vi "Teeth Force Torque2___C.vi"() -> ()   [LabVIEW 2011]
doc: "Reads force and torque values from multiple ATI transducers."
uses:
  <vilib>/DAQmx/read.llb/DAQmx Read (Analog 2D DBL NChan NSamp).vi
  <vilib>/DAQmx/miscellaneous.llb/DAQmx Fill In Error Info.vi
  <vilib>/Analysis/baseanly.llb/A x Vector.vi
  <vilib>/Analysis/NI_AALBase.lvlib
  Program Files/MATLAB/R2010a/work/OSIM2/lib/OSIM_itf1.dll
panel:
  out "Average Voltages":dbl[][](array[numeric]) format="%#_3g"
  out "exiting":bool
  in  "stop":bool
  in  "Calibration File Directory:":path=path "C:/Documents and Settings/ortholab/Desktop/Load Cells Calibration Files Feb 2015"
  in  "Bias Transducer":bool[](array[boolean])=[FALSE, FALSE, FALSE, FALSE, FALSE, FALSE, FALSE, FALSE, FALSE, FALSE, FALSE, FALSE, FALSE, FALSE]
  in  "Calibration Files":string[](array[string])=["ft16995.cal", "ft6798.cal", "ft6799.cal", "ft6800.cal", "ft13847.cal", "ft6802.cal", "ft16994.cal", "ft6804.cal", "ft6805.cal", "ft5393.cal", "ft6807.cal", "ft6808.cal", "ft10276.cal", "ft13846.cal"]
  in  "Filename":path
  in  "Bias All":bool
  in  "Save Data Point":bool
  in  "Samples to Read at a time":i32=50
  out "Cal F/T Values":dbl[][](array[numeric])
  # "OSIM"
  # "Fx"
  # "Fy"
  # "Fz"
  # "Ty"
  # "Tz"
  # "Tx"
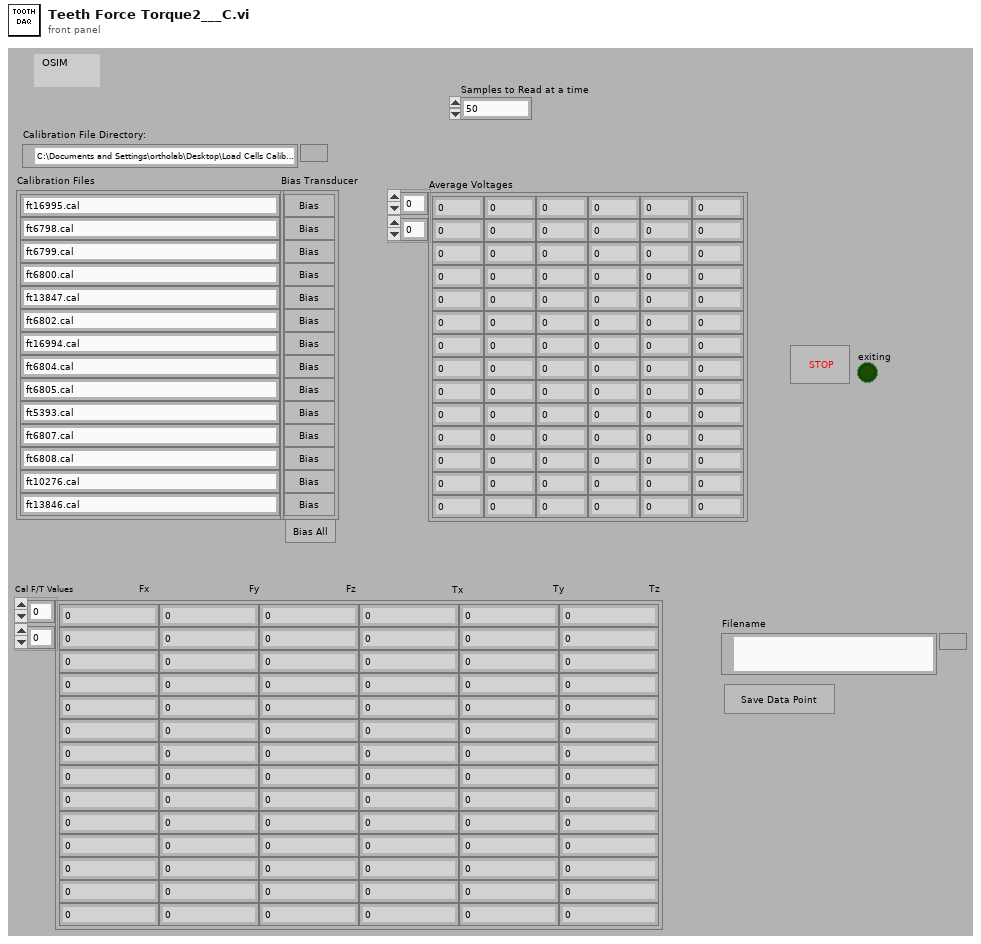
[diagram p1: front panel]
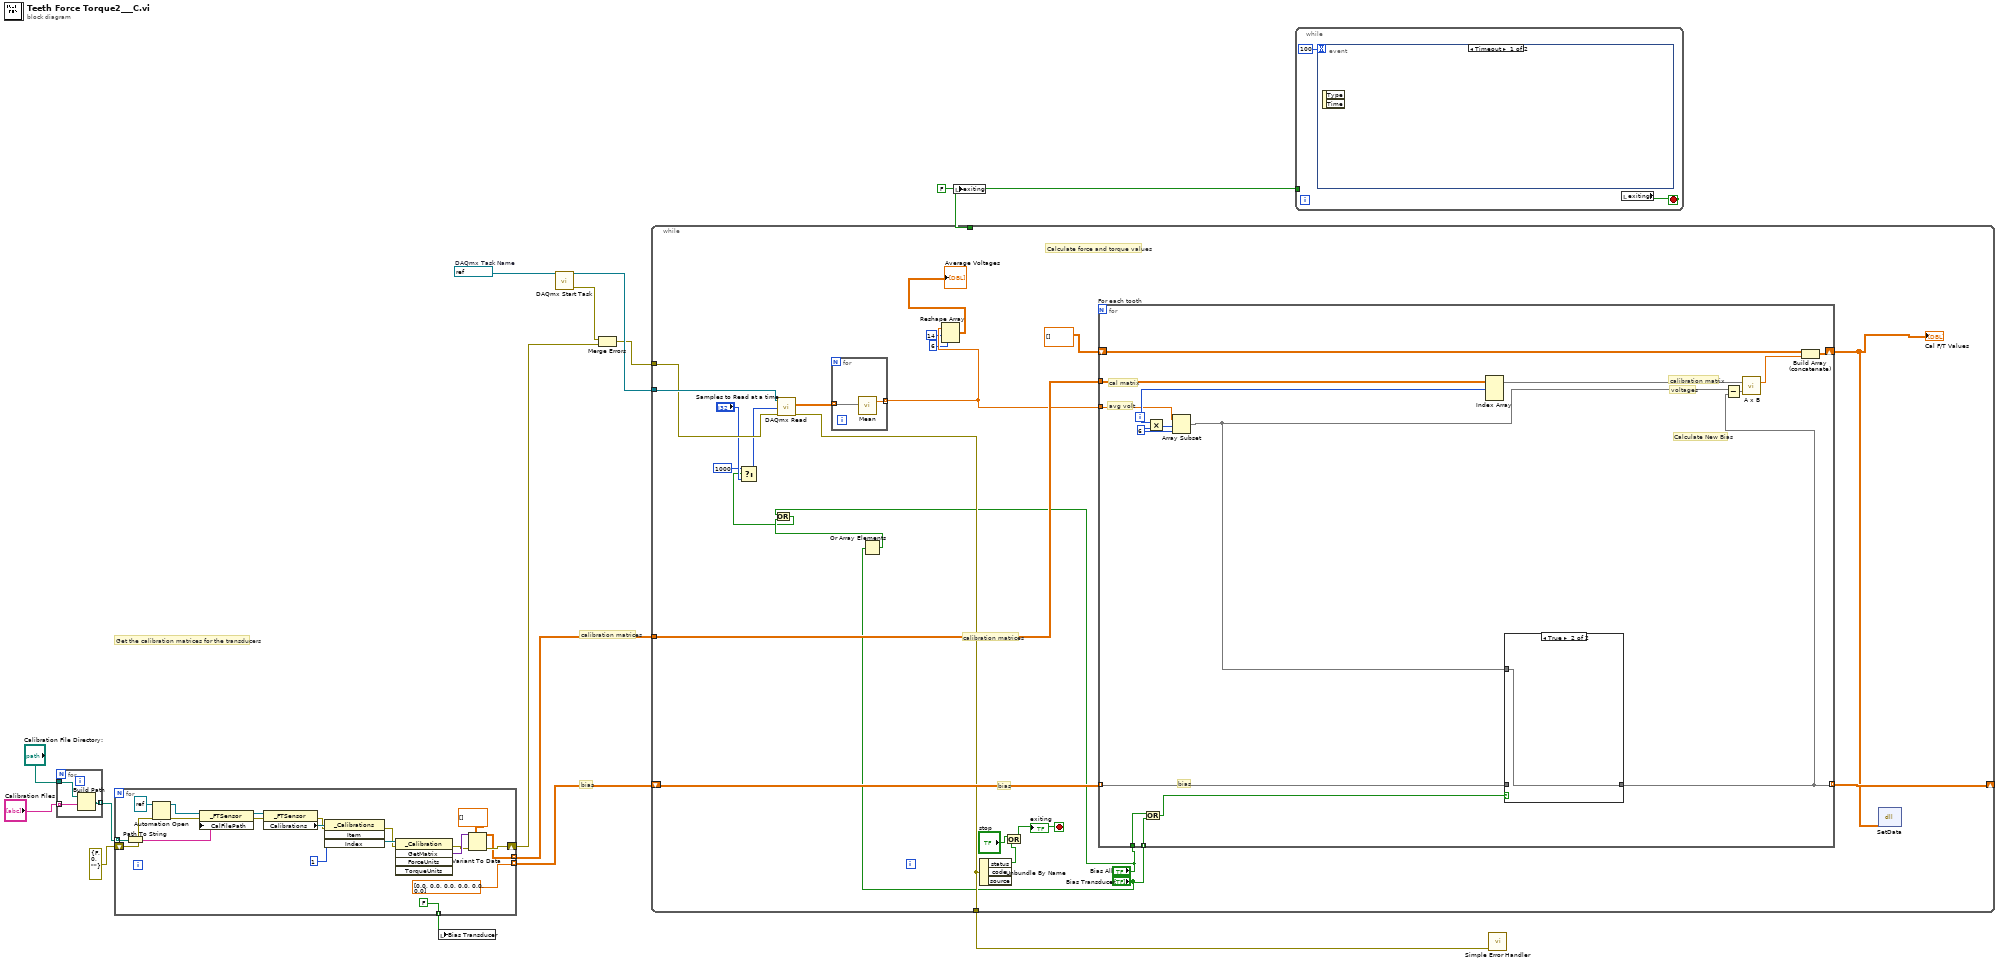
[diagram p0: block diagram]
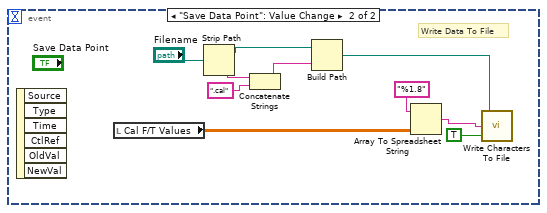
[diagram p2: hidden frame]
diagram:
  w1 = FALSE ("exiting")
  w2 = refnum<k21> "TEETH1"  # DAQmx Task Name
  # "bias"
  # "calibration matrices"
  # "Get the calibration matrices for the transducers"
  n1 = for {
    tunnel: "Calibration File Directory:" -> [w17]
    tunnel: [w16] -> w4 mode=indexing
    tunnel: "Calibration Files" -> [w15] mode=indexing
    n2 = Build Path(base path=w17, name or relative path=w15) -> (appended path=w16:path)
  }
  n3 = for {
    tunnel: w4 -> [w34] mode=indexing
    shift-right: [w25] -> w10
    shift-left: errorcluster {"status"=FALSE, "code"=0, "source"=""} ("error out") -> [w22]
    tunnel: [FALSE] -> w12 mode=indexing
    tunnel: [sgl[] [0.0, 0.0, 0.0, 0.0, 0.0, 0.0]] -> w11 mode=indexing
    tunnel: [w18] -> w7 mode=indexing
    n4 = Path To String(path=w34) -> (string=w33:string)
    n5 = Automation Open(error in (no error)=w22, Automation Refnum=refnum<k7> refnum ("ATIDAQFT._FTSensor")) -> (Automation Refnum=w23:refnum<k7>, error out=w21:errorcluster)  [unwired: 2 in]
    n6 = property class="_FTSensor"(reference=w23, error in=w21, "CalFilePath"=w33) -> (reference out=w35:refnum<k7>, error out=w29:errorcluster)
    n7 = property class="_FTSensor"(reference=w35, error in=w29) -> (error out=w28:errorcluster, "Calibrations"=w37:refnum<k7>)  [unwired: 1 out]
    n8 = invoke class="_Calibrations" method="Item"(reference=w37, error in=w28, "Index"=1) -> (error out=w27:errorcluster, "Item"=w32:refnum<k7>)  [unwired: 1 in, 2 out]
    n9 = invoke class="_Calibration" method="GetMatrix"(reference=w32, error in=w27) -> (error out=w26:errorcluster, "GetMatrix"=w31:variant)  [unwired: 3 in, 3 out]
    n10 = Variant To Data(error in=w26, type=sgl[][] [], Variant=w31) -> (data=w18:sgl[][], error out=w25:errorcluster)
  }
  n11 = local write "Bias Transducer"(w12) -> ()
  n12 = call <vilib>:"DAQmx Start Task.vi"("task/channels in"=w2) -> ("task out"=w14:refnum<k21>, "error out"=w9:errorcluster)  [unwired: 13 in]
  n13 = Merge Errors(w9, w10) -> (w8:errorcluster)
  n14 = while {
    tunnel: w14 -> [w60]
    tunnel: w7 -> [w59]
    shift-right: [w57] -> _
    shift-left: w11 -> [w58]
    tunnel: w8 -> [w50]
    tunnel: [w56] -> w6
    tunnel: w1 -> [_]
    stop <- w53 stop-if-true
    # "bias"
    # "calibration matrices"
    # "Calculate force and torque values"
    n15 = Or Array Elements(Boolean array="Bias Transducer") -> (logical OR=w44:bool)
    n16 = Or(x="Bias All", y=w44) -> (x .or. y?=w42:bool)
    n17 = Select(t=1000, s=w42, f="Samples to Read at a time") -> (s? t:f=w48:i32)
    n18 = call-poly <vilib>:"DAQmx Read.vi"("task/channels in"=w60, "number of samples per channel"=w48, "error in"=w50) -> ("data"=w52:dbl[][], "error out"=w56:errorcluster)  [unwired: 10 in, 1 out]
    n19 = for {
      tunnel: w52 -> [w80] mode=indexing
      tunnel: [w79] -> w41 mode=indexing
      n20 = call <vilib>:"Mean.vi"("X"=w80) -> ("mean"=w79:dbl)  [unwired: 1 out]
    }
    n21 = Reshape Array(w41, 14 ("dimension size"), 6 ("dimension size")) -> (→"Average Voltages":dbl[][])
    n22 = Unbundle By Name(w56) -> ("status"=w54:bool)  [unwired: 2 out]
    n23 = Compound Arithmetic op=OR("stop", w54) -> (w53:bool)
    "exiting" <- w53
    n24 = for "For each tooth" {
      tunnel: w59 -> [w72]
      tunnel: w58 -> [w75] mode=indexing
      tunnel: "Bias Transducer" -> [w76] mode=indexing
      tunnel: [w74] -> w57 mode=indexing
      tunnel: "Bias All" -> [w73]
      shift-right: [w69] -> w49
      shift-left: sgl[][] [] -> [w70]
      tunnel: w41 -> [w64]
      i -> [w71]
      w67 = 6
      # "cal matrix"
      # "avg volt"
      # "bias"
      # "voltages"
      # "calibration matrix"
      # "Calculate New Bias"
      n25 = Or(x=w73, y=w76) -> (x .or. y?=w62:bool)
      n26 = Multiply(x=w71, y=w67) -> (x*y=w68:i32)
      n27 = Array Subset(array=w64, index=w68, length=w67) -> (w61:dbl[])
      n28 = Index Array(array=w72, index (dim 0)=w71) -> (element=w65:sgl[][])  [unwired: 2 in]
      n29 = case shown="True" w62 {
        tunnel: [w77 w78] -> w74
        tunnel: w75 -> [w77 _]
        tunnel: w61 -> [_ w78]
        frame False {
        }
        frame True {
        }
      }
      n30 = Subtract(x=w61, y=w74) -> (x-y=w66:dbl[])
      n31 = call-poly <vilib>:"A x B.vi"("Vector"=w66, "A"=w65) -> ("A x Vector"=w63:dbl[])  [unwired: 1 out]
      n32 = Build Array (concatenate)(w70, w63) -> (w69:dbl[][])
    }
    "Cal F/T Values" <- w49
    n33 = dll-call lib="C:/Program Files/MATLAB/R2010a/work/OSIM2/lib/OSIM_itf1.dll" fn="SetData" ("shell32.dll:SHCreateStdEnumFmtEtc")("arg1"=w49) -> ()  [unwired: 5 in, 2 out]
  }
  n34 = local write "exiting"(w1) -> ()
  n35 = while {
    tunnel: w1 -> [_]
    stop <- w82 stop-if-true
    n36 = event shown="[0] Timeout" {
      selector: _ -> [_ _]
      dyn-events: _ -> [_ _]
      timeout: 100 -> [_ _]
      event Timeout {
        n37 = event-data() -> ()  [unwired: 1 in, 2 out]
      }
      event "Save Data Point": Value Change {
        # "Write Data To File"
        n38 = event-data() -> ()  [unwired: 1 in, 6 out]
        n39 = local read "Cal F/T Values"() -> (w83:dbl[][])
        n40 = Strip Path(path="Filename") -> (stripped path=w85:path, name=w87:string)
        n41 = Concatenate Strings(w87, ".cal" ("string")) -> (w86:string)
        n42 = Build Path(base path=w85, name or relative path=w86) -> (appended path=w84:path)
        n43 = Array To Spreadsheet String(array=w83, 3:"%1.8" ("format string")) -> (spreadsheet string=w90:string)  [unwired: 1 in]
        n44 = call <vilib>:"Write Characters To File.vi"("append to file? (new file:F)"=TRUE, "character string"=w90, "file path (dialog if empty)"=w84) -> ()  [unwired: 2 in, 1 out]
      }
    }
    n45 = local read "exiting"() -> (w82:bool)
  }
  n46 = call <vilib>:"Simple Error Handler.vi"("error in (no error)"=w6) -> ()  [unwired: 4 in, 5 out]
